vi "Query IO.vi"(8 "error in":errorcluster, 11 "ProXR in":refnum<class "ProXR.lvclass">) -> (0 "error out":errorcluster, 1 "Port Array":u8[](array[numeric]), 2 "Boolean Array":bool[](array[boolean]), 3 "ProXR out":refnum<class "ProXR.lvclass">)   [LabVIEW 2019, in "ProXR.lvlib" / "ProXR.lvclass"]
doc: "This method must be overridden by the child class.\n\nThis should read the status at the output of the device and return a weform capture of the named signal states."
uses:
  Library/ProXR.lvclass
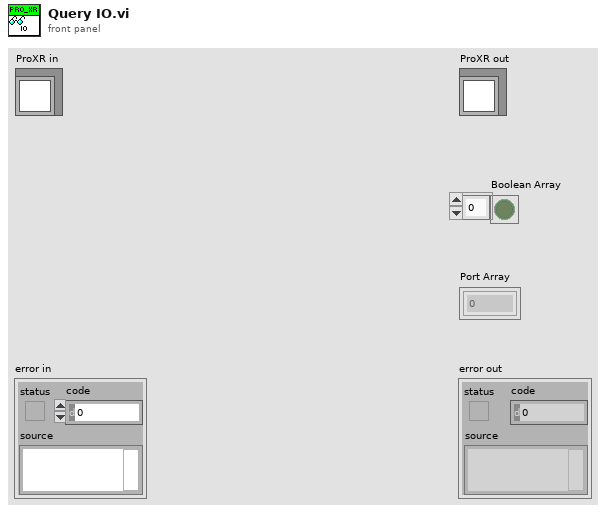
[diagram p1: front panel]
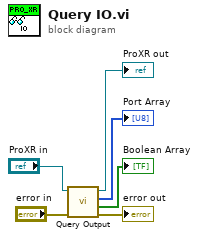
[diagram p0: block diagram]
diagram:
  n1 = call "Query Output.vi"("error in"="error in", "ProXR_IO in"="ProXR in") -> ("error out"=→"error out":errorcluster, "Digital Out"=→"Boolean Array":bool[], "Query All Banks"=→"Port Array":u8[], "ProXR_IO out"=→"ProXR out":refnum<class "ProXR.lvclass">)  [unwired: 6 in]
